vi "p02  prueba.vi"() -> ()   [LabVIEW 2020]
panel:
  out "Image":T1(plugin-control)
  in  "Path":path
  out "new picture":picture
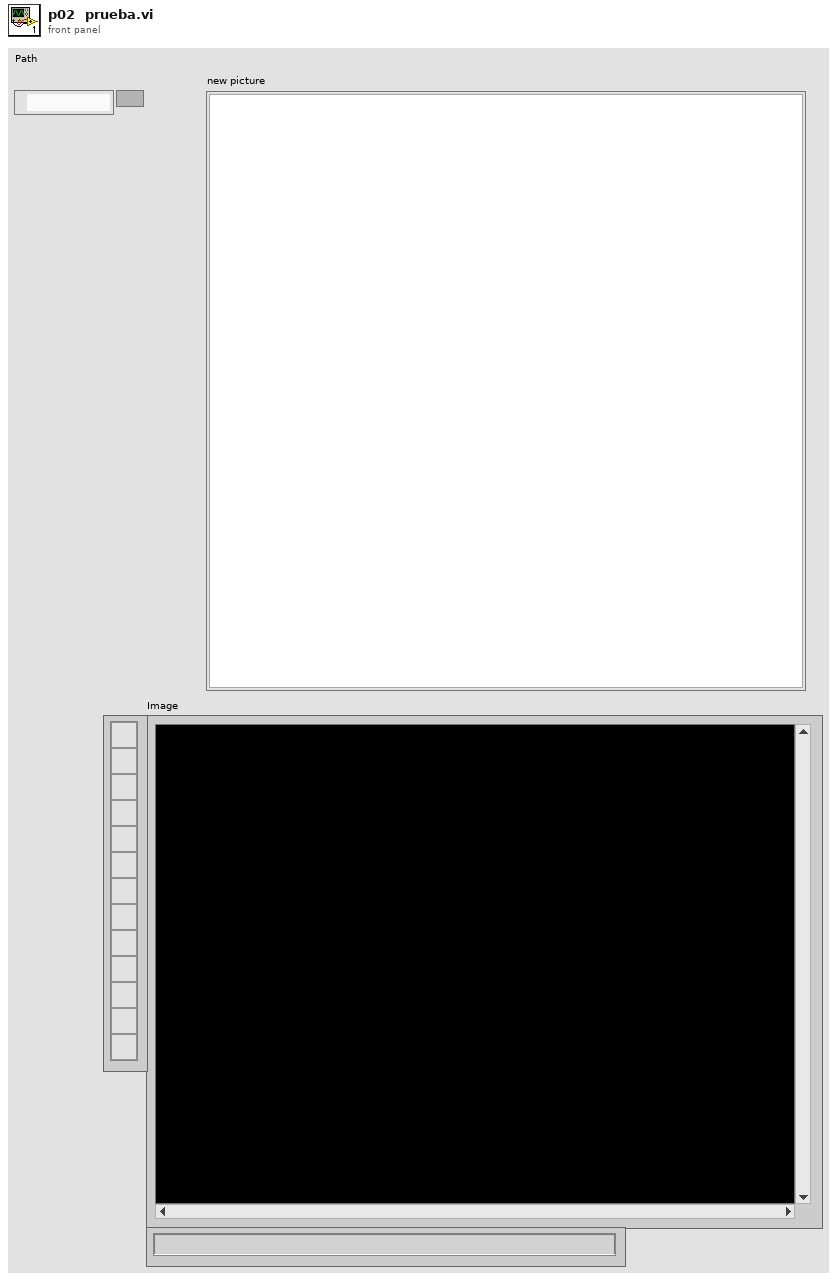
[diagram p1: front panel]
types:
  T1 = typedef "IMAQ Image.ctl" = refnum<image>
  T2 = typedef "imagedata.ctl" = cluster{"image type":i32, "image depth":i32, "image":u8[], "mask":u8[], "colors":u32[], "Rectangle":cluster{"left":i16, "top":i16, "right":i16, "bottom":i16}}
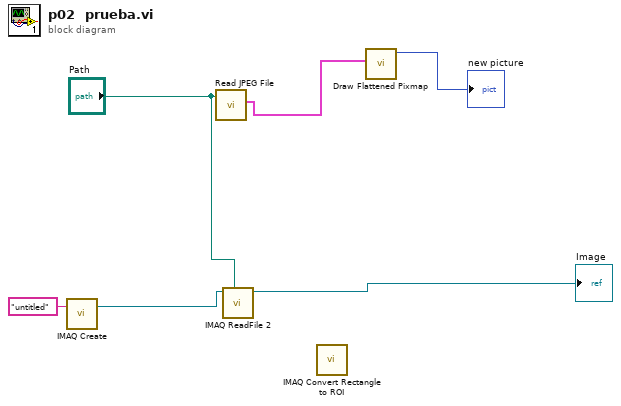
[diagram p0: block diagram]
diagram:
  n1 = call "IMAQ Create"("Image Name"="untitled") -> ("New Image"=w3:T1)  [unwired: 4 in, 1 out]
  n2 = call <vilib>:"Read JPEG File.vi"("path to JPEG file"="Path") -> ("image data"=w5:T2)  [unwired: 8 in, 2 out]
  n3 = call "IMAQ ReadFile 2"("File Path"="Path", "Image"=w3) -> ("Image Out"=→"Image":T1)  [unwired: 5 in, 4 out]
  n4 = call "IMAQ Convert Rectangle to ROI"() -> ()  [unwired: 9 in, 2 out]
  n5 = call <vilib>:"Draw Flattened Pixmap.vi"("image data"=w5) -> ("new picture"=→"new picture":picture)  [unwired: 8 in]
